vi "PH_ImageStatistician.PC Select Data.vi"(0 "i ref in":refnum<vi>, 1 "Stat or Trend":bool, 2 "Data 1":T1 items=["nothing ", "FWHM Major Trace", "FWHM Minor Trace", "Gaussian Fit Order Major Trace", "Gaussian Fit Order Minor Trace", "99% Diameter Major Trace", "99% Diameter Minor Trace", "Theta", "Delta", "Major Diameter", "Minor Diameter", "Azimuth Angle", "Azi Angle rel to Major?", "Ellipticity", "Center of gravity - x", "Center of gravity - y", "Energy"], 3 "Data 2":T1 items=["nothing ", "FWHM Major Trace", "FWHM Minor Trace", "Gaussian Fit Order Major Trace", "Gaussian Fit Order Minor Trace", "99% Diameter Major Trace", "99% Diameter Minor Trace", "Theta", "Delta", "Major Diameter", "Minor Diameter", "Azimuth Angle", "Azi Angle rel to Major?", "Ellipticity", "Center of gravity - x", "Center of gravity - y", "Energy"], 4 "Data 3":T1 items=["nothing ", "FWHM Major Trace", "FWHM Minor Trace", "Gaussian Fit Order Major Trace", "Gaussian Fit Order Minor Trace", "99% Diameter Major Trace", "99% Diameter Minor Trace", "Theta", "Delta", "Major Diameter", "Minor Diameter", "Azimuth Angle", "Azi Angle rel to Major?", "Ellipticity", "Center of gravity - x", "Center of gravity - y", "Energy"], 5 "error in (no error)":errorcluster) -> (14 "i ref out":refnum<vi>, 19 "error out":errorcluster)   [LabVIEW 2014, in "PH_ImageStatistician.lvlib"]
doc: "This VI sets attributes and some GUI elements. It contains the get data to modify / set modified data -vis, handle with care!"
uses:
  PH_ImageStatistician.lvlib
  PH_ImageStatistician.select Data.ctl
  PH_Basics/PH_Common/PH_Common.lvlib
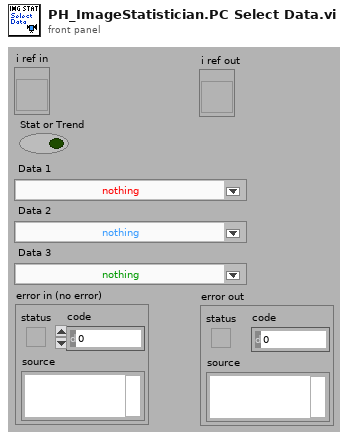
[diagram p1: front panel]
types:
  T1 = typedef "PH_ImageStatistician.lvlib/PH_ImageStatistician.select Data.ctl" = u16
  T2 = typedef "PH_ImageStatistician.lvlib/PH_ImageStatistician.i attribute.ctl" = cluster{"GUI Refs ":cluster{"Status":refnum<vi>, "Result Graph":refnum<vi>, "Mean Data 1":refnum<vi>, "Std Dev Data 1":refnum<vi>, "Mean Data 2":refnum<vi>, "Std Dev Data 2":refnum<vi>, "Mean Data 3":refnum<vi>, "Std Dev Data 3":refnum<vi>, "Dummy Mean":refnum<vi>, "Dummy Std Dev":refnum<vi>, "Export Data":refnum<vi>, "Data 1":refnum<vi>, "Data 2":refnum<vi>, "Data 3":refnum<vi>, "Stat or Trend":refnum<vi>, "Delete":refnum<vi>, "Operator":refnum<vi>, "Start":refnum<vi>}, "Operator":string, "Data":T3[], "Stat or Trend":bool, "Data 1":T1, "Data 2":T1, "Data 3":T1, "Start":bool, "Datasets strored":i32, "Dataarray Size":i32}
  T3 = typedef "PH_ImageStatistician.lvlib/PH_ImageStatistician.Statistician Data.ctl" = cluster{"Snapshot Time":dbl, "Maj FWHM":dbl, "Min FWHM":dbl, "Maj Fit Order":dbl, "Min Fit Order":dbl, "99% Diam Maj Trace":dbl, "99% Diam Min Trace":dbl, "Theta":dbl, "Delta":dbl, "Maj Diam":dbl, "Min Diam":dbl, "Azimuth Angle":dbl, "Azi Angle rel to major?":dbl, "Ellipticity":dbl, "CoG - X":dbl, "CoG - Y":dbl, "Energy":dbl, "Energy Cal - no mJ":dbl, "Lin Cal - no mm or mrad":dbl, "Lin Cal Factor":dbl}
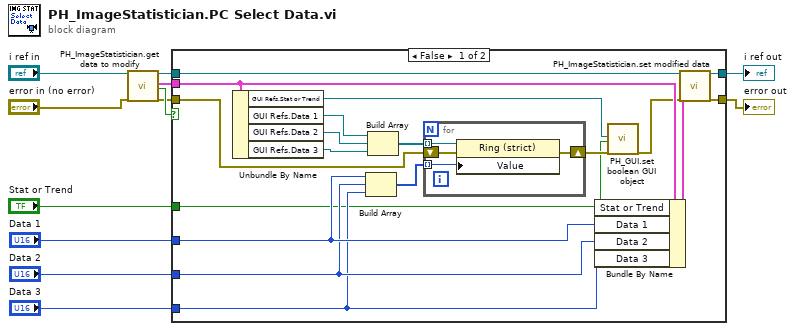
[diagram p0: block diagram]
diagram:
  n1 = call "PH_ImageStatistician.get data to modify.vi"("i ref in"="i ref in", "error in (no error)"="error in (no error)") -> ("i ref out"=w7:refnum<vi>, "i attribute"=w11:T2, "timed out"=w10:bool, "error out"=w6:errorcluster)  [unwired: 14 in]
  n2 = case shown="False" w10 {
    tunnel: w6 -> [w20 w35]
    tunnel: w7 -> [w30 w36]
    tunnel: [w29 w36] -> w8
    tunnel: [w28 w35] -> w9
    tunnel: w11 -> [w26 _]
    tunnel: "Stat or Trend" -> [w13 _]
    tunnel: "Data 1" -> [w19 _]
    tunnel: "Data 2" -> [w18 _]
    tunnel: "Data 3" -> [w17 _]
    frame False {
      n3 = Unbundle By Name(w26) -> ("GUI Refs.Stat or Trend"=w14:refnum<vi>, "GUI Refs.Data 1"=w24:refnum<vi>, "GUI Refs.Data 2"=w23:refnum<vi>, "GUI Refs.Data 3"=w22:refnum<vi>)
      n4 = Build Array(w19, w18, w17) -> (w16:T1[])
      n5 = Build Array(w24, w23, w22) -> (w21:refnum<vi>[])
      n6 = for {
        tunnel: w21 -> [w32] mode=indexing
        shift-right: [w33] -> w25
        shift-left: w20 -> [w34]
        tunnel: w16 -> [w31] mode=indexing
        n7 = property class="Ring (strict)"(reference=w32, error in=w34, "Value"=w31) -> (error out=w33:errorcluster)  [unwired: 1 out]
      }
      n8 = Bundle By Name(cluster=w26, "Stat or Trend"=w13, "Data 1"=w19, "Data 2"=w18, "Data 3"=w17) -> (w27:T2)
      n9 = call "PH_GUI.set boolean GUI object.vi"("Boolean Knob GUI Ref"=w14, "Value"=w13, "error in (no error)"=w25) -> ("error out"=w15:errorcluster)  [unwired: 16 in]
      n10 = call "PH_ImageStatistician.set modified data.vi"("i ref in"=w30, "i attribute"=w27, "error in (no error)"=w15) -> ("i ref out"=w29:refnum<vi>, "error out"=w28:errorcluster)  [unwired: 15 in]
    }
    frame True {
    }
  }
  "error out" <- w9
  "i ref out" <- w8
